vi "Begin.vi"(11 "Image Size":T1=enum."160x120") -> (0 "error out":errorcluster)   [LabVIEW 2012]
doc: "Called before other user functions, this VI is expected to open initial I/O refnums, load in file data, and do all program initialization. Notice that the <B>error out</B> terminal is simply used for data flow. Wiring it to other structures or subVIs ensures that this VI runs first."
uses:
  <vilib>/Rock Robotics/WPI/Camera/WPI_CameraImageSize.ctl
  <vilib>/Rock Robotics/WPI/DriverStation/WPI_DriverStationRobotMode2.ctl
  <vilib>/Rock Robotics/WPI/Joystick/WPI_JoystickDeviceEnum.ctl
  <vilib>/Rock Robotics/WPI/CAN/Jaguar/SubVIs/WPI_CANJaguar_ControlMode.ctl
  <vilib>/Rock Robotics/WPI/CAN/Jaguar/SubVIs/WPI_CANJaguar_SpeedReference.ctl
  <vilib>/Rock Robotics/WPI/CAN/Jaguar/SubVIs/WPI_CANJaguar_BrakeCoastMode.ctl
  <vilib>/Rock Robotics/WPI/CAN/Jaguar/SubVIs/WPI_CANJaguar_PositionReference.ctl
  <vilib>/Rock Robotics/SystemInterfaces/Typedef/FPGA_TypedefDigitalModule.ctl
  <vilib>/Rock Robotics/SystemInterfaces/DIO/FPGA_DIOChannel.ctl
  <vilib>/Rock Robotics/SystemInterfaces/Typedef/FPGA_TypedefSolenoidModule.ctl
  <vilib>/Rock Robotics/WPI/Solenoid/WPI_SolenoidChannel.ctl
  <vilib>/Rock Robotics/SystemInterfaces/DIO/FPGA_DIORelayChannel.ctl
  Robot Global Data.vi
  <vilib>/Rock Robotics/WPI/MotorControl/WPI_MotorControlOpenCANJaguar.vi
  <vilib>/Rock Robotics/WPI/Solenoid/WPI_SolenoidOpenSingle.vi
  <vilib>/Rock Robotics/WPI/Compressor/WPI_CompressorGetSetRefNum.vi
  <vilib>/Rock Robotics/WPI/Camera/WPI_CameraWhite Balance Values.ctl
  <vilib>/Rock Robotics/WPI/Camera/WPI_CameraExposure Values.ctl
  <vilib>/Rock Robotics/WPI/Camera/WPI_CameraFrameRate.ctl
  <vilib>/Rock Robotics/WPI/RobotDrive/WPI_RobotDriveOpen4MotorWithCANJaguar.vi
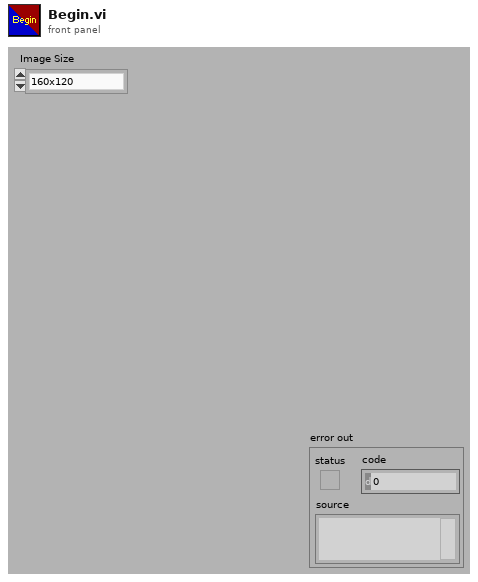
[diagram p1: front panel]
types:
  T1 = typedef "WPI_CameraImageSize.ctl" = enum16{"640x480", "320x240", "160x120"}
  T2 = typedef "FPGA_DIORelayChannel.ctl" = enum8{"Relay 1", "Relay 2", "Relay 3", "Relay 4", "Relay 5", "Relay 6", "Relay 7", "Relay 8", "Invalid"}
  T3 = typedef "WPI_SolenoidChannel.ctl" = enum8{"Solenoid 1", "Solenoid 2", "Solenoid 3", "Solenoid 4", "Solenoid 5", "Solenoid 6", "Solenoid 7", "Solenoid 8", "Invalid"}
  T4 = typedef "FPGA_TypedefSolenoidModule.ctl" = enum16{"Solenoid Module 1", "Solenoid Module 2"}
  T5 = typedef "FPGA_DIOChannel.ctl" = enum8{"DIO 1", "DIO 2", "DIO 3", "DIO 4", "DIO 5", "DIO 6", "DIO 7", "DIO 8", "DIO 9", "DIO 10", "DIO 11", "DIO 12", "DIO 13", "DIO 14", "Invalid"}
  T6 = typedef "FPGA_TypedefDigitalModule.ctl" = enum16{"Digital Module 1", "Digital Module 2"}
  T7 = typedef "WPI_JoystickDeviceEnum.ctl" = enum16{"USB 1", "USB 2", "USB 3", "USB 4", "Kinect 1", "Kinect 2"}
  T8 = typedef "WPI_CANJaguar_PositionReference.ctl" = u8
  T9 = typedef "WPI_CANJaguar_BrakeCoastMode.ctl" = enum8{"Jumper", "Brake", "Coast"}
  T10 = typedef "WPI_CANJaguar_ControlMode.ctl" = enum8{"Percent VBus", "Current", "Speed", "Position", "Voltage"}
  T11 = typedef "WPI_CANJaguar_SpeedReference.ctl" = u8
  T12 = typedef "WPI_DriverStationRobotMode2.ctl" = enum16{"Autonomous Disabled", "Autonomous Enabled", "Teleop Disabled", "Teleop Enabled", "Timeout", "Finish", "Test Disabled", "Test Enabled"}
  T13 = typedef "WPI_JoystickDevRef.ctl" = cluster{"Device":T7}
  T14 = typedef "WPI_SolenoidDevRef.ctl" = cluster{"DevStatus":errorcluster, "Solenoid Module":T4, "Forward Solenoid Channel":T3, "Reverse Solenoid Channel":T3}
  T15 = typedef "WPI_DigitalInputDevRef.ctl" = cluster{"DevStatus":errorcluster, "DIO Channel":T5, "Digital Module":T6}
  T16 = typedef "WPI_CompressorDevRef.ctl" = cluster{"DevStatus":errorcluster, "DigitalInputDevRef":T15, "RelayDevRef":T17}
  T17 = typedef "WPI_RelayDevRef.ctl" = cluster{"DevStatus":errorcluster, "Relay Channel":T2, "Digital Module":T6, "Relay Direction":T18}
  T18 = typedef "WPI_RelayDirection.ctl" = enum16{"Both directions", "Forward only", "Reverse only"}
  T19 = typedef "WPI_SerialPortRef.ctl" = cluster{"DevStatus":errorcluster, "Serial Port Name":refnum<visa-resource-name>}
  T20 = typedef "WPI_CameraFrameRate.ctl" = u32
  T21 = typedef "WPI_CameraExposure Values.ctl" = enum16{"Auto", "Flicker-free 50 Hz", "Flicker-free 60 Hz", "Hold current"}
  T22 = typedef "WPI_CameraWhite Balance Values.ctl" = enum16{"Auto", "Fixed indoor", "Fixed outdoor 1", "Fixed outdoor 2", "Fixed fluorescent 1", "Fixed fluorescent 2", "Hold current"}
  T23 = typedef "WPI_CameraDevRef.ctl" = cluster{"Camera Address":string, "CameraStatus":errorcluster, "Acquire Image Notifier":refnum<notifier>}
  T24 = typedef "WPI_MotorControlDeviceRef.ctl" = cluster{"DeviceStatus":errorcluster, "Type":enum16{"PWM", "CAN"}, "PWM":cluster{"Digital Module":T6, "PWM Channel":T25, "DeadBand":T26}, "CAN":cluster{"Device Number":u8, "Control Mode":T10, "Semaphore":T27, "Max Vout":dbl}, "Invert":bool, "TransformRef":T28, "InvTransformRef":T28}
  T25 = typedef "FPGA_DIOPWMChannel.ctl" = enum8{"PWM 1", "PWM 2", "PWM 3", "PWM 4", "PWM 5", "PWM 6", "PWM 7", "PWM 8", "PWM 9", "PWM 10", "Invalid"}
  T26 = typedef "WPI_PWMDeadband.ctl" = cluster{"Name":string, "maxPositivePwm":i32, "minPositivePwm":i32, "centerPwm":i32, "maxNegativePwm":i32, "minNegativePwm":i32, "angularRange":u16}
  T27 = typedef "Semaphore RefNum" = refnum<k1>
  T28 = typedef "WPI_PWMTransform_ConPane.ctl" = refnum<vi>
  T29 = typedef "WPI_RobotDriveDevRef.ctl" = cluster{"DevStatus":errorcluster, "Motors[]":T24[], "Square Inputs":bool, "Max Output":dbl, "Isochronous":bool}
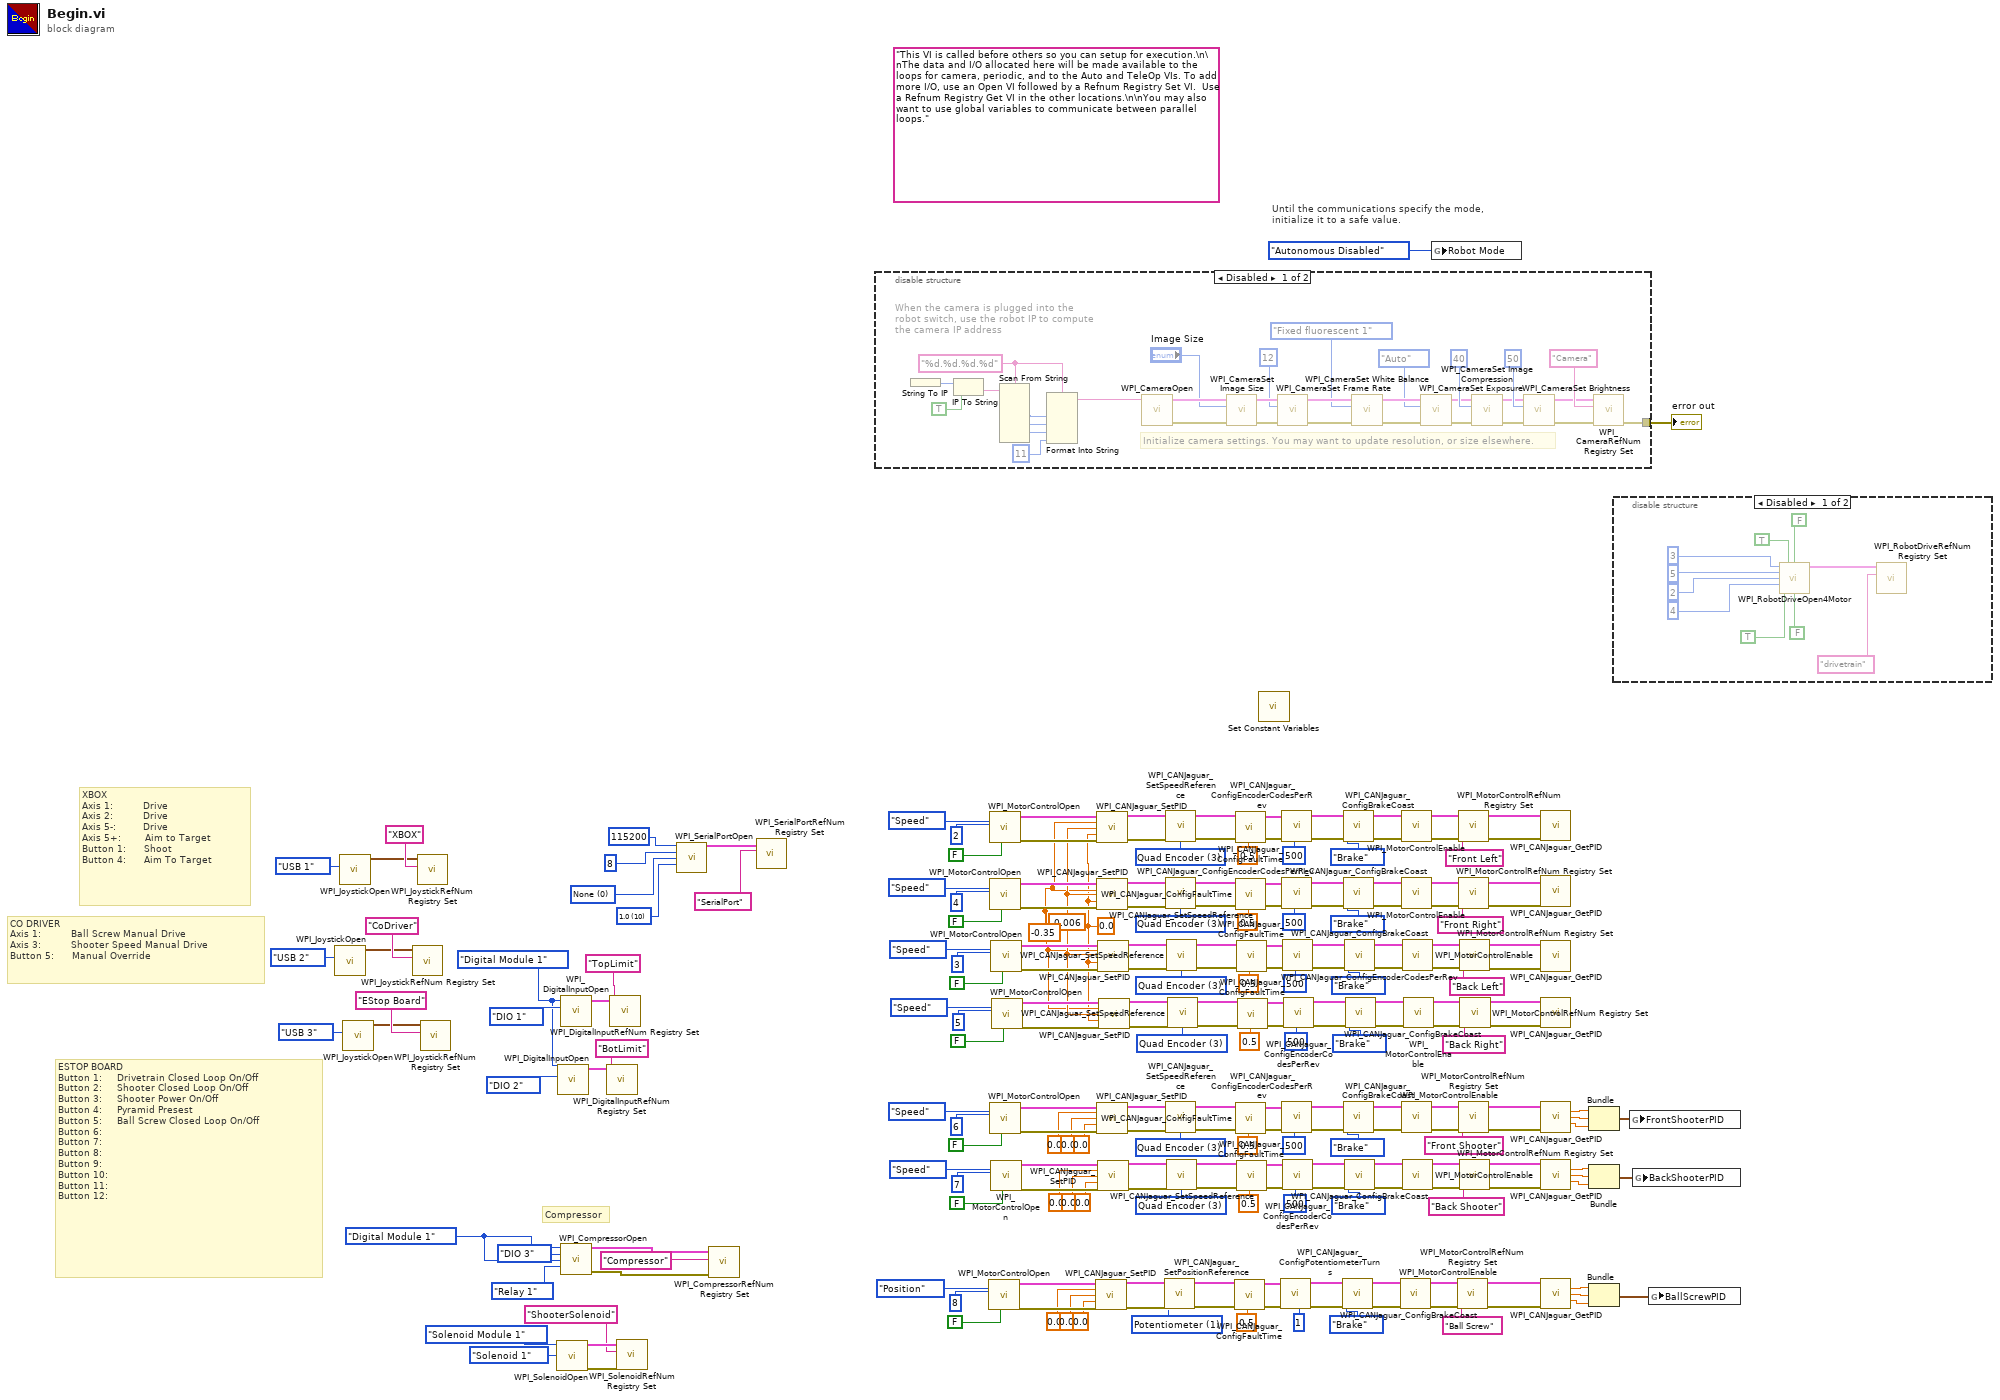
[diagram p0: block diagram]
diagram:
  w2 = FPGA_TypedefDigitalModule."Digital Module 1" ("Pressure Switch Digital Module (Module 1)")
  w12 = FPGA_TypedefDigitalModule."Digital Module 1" ("Digital Module (Module 1)")
  w54 = T8 1 items=["Quad Encoder"=0, "Potentiometer"=1, "None"=255] ("Position Reference")
  w93 = T11 3 items=["Encoder"=0, "Inv Encoder"=2, "Quad Encoder"=3, "None"=255] ("Speed Reference")
  w118 = T11 3 items=["Encoder"=0, "Inv Encoder"=2, "Quad Encoder"=3, "None"=255] ("Speed Reference")
  w140 = T11 3 items=["Encoder"=0, "Inv Encoder"=2, "Quad Encoder"=3, "None"=255] ("Speed Reference")
  w162 = T11 3 items=["Encoder"=0, "Inv Encoder"=2, "Quad Encoder"=3, "None"=255] ("Speed Reference")
  w184 = T11 3 items=["Encoder"=0, "Inv Encoder"=2, "Quad Encoder"=3, "None"=255] ("Speed Reference")
  w20 = -0.35 ("P")
  w21 = -0.006 ("I")
  w19 = 0.0 ("D")
  w206 = T11 3 items=["Encoder"=0, "Inv Encoder"=2, "Quad Encoder"=3, "None"=255] ("Speed Reference")
  w219 = u16 10 items=["1.0"=10, "1.5"=15, "2.0"=20] ("Stop Bits")
  w220 = u16 0 items=["None", "Odd", "Even", "Mark", "Space"] ("Parity")
  (unwired) "This VI is called before others so you can setup for execution.\n\nThe data and I/O allocated here will be made available to the loops for camera, periodic, and to the Auto and TeleOp VIs. To add more I/O, use an Open VI followed by a Refnum Registry Set VI.  Use a Refnum Registry Get VI in the other locations.\n\nYou may also want to use global variables to communicate between parallel loops."
  # "Compressor"
  # "CO DRIVER\nAxis 1:          Ball Screw Manual Drive\nAxis 3:          Shooter Speed Manual Drive\nButton 5:      Manual Override"
  # "XBOX\nAxis 1:          Drive\nAxis 2:          Drive\nAxis 5-:         Drive\nAxis 5+:        Aim to Target\nButton 1:      Shoot\nButton 4:      Aim To Target"
  # "ESTOP BOARD\nButton 1:     Drivetrain Closed Loop On/Off\nButton 2:     Shooter Closed Loop On/Off\nButton 3:     Shooter Power On/Off\nButton 4:     Pyramid Presest\nButton 5:     Ball Screw Closed Loop On/Off\nButton 6:     \nButton 7:\nButton 8:\nButton 9:\nButton 10:\nButton 11:\nButton 12:"
  # "Until the communications specify the mode,\ninitialize it to a safe value."
  n1 = call <vilib>:"WPI_JoystickOpen.vi"("JoystickDevice"=WPI_JoystickDeviceEnum."USB 2") -> ("JoystickDevRef"=w26:T13)  [unwired: 10 in]
  n2 = call <vilib>:"WPI_JoystickOpen.vi"("JoystickDevice"=WPI_JoystickDeviceEnum."USB 1") -> ("JoystickDevRef"=w225:T13)  [unwired: 10 in]
  n3 = call <vilib>:"WPI_JoystickOpen.vi"("JoystickDevice"=WPI_JoystickDeviceEnum."USB 3") -> ("JoystickDevRef"=w23:T13)  [unwired: 10 in]
  n4 = call <vilib>:"WPI_JoystickRefNum Registry Set.vi"("refnum name"="CoDriver", "JoystickDevRef"=w26) -> ()  [unwired: 8 in, 2 out]
  n5 = call <vilib>:"WPI_JoystickRefNum Registry Set.vi"("refnum name"="XBOX", "JoystickDevRef"=w225) -> ()  [unwired: 8 in, 2 out]
  n6 = call <vilib>:"WPI_JoystickRefNum Registry Set.vi"("refnum name"="EStop Board", "JoystickDevRef"=w23) -> ()  [unwired: 8 in, 2 out]
  n7 = call-poly <vilib>:"WPI_SolenoidOpen.vi"("Solenoid Channel"=WPI_SolenoidChannel."Solenoid 1", "Solenoid Module (Module 1)"=FPGA_TypedefSolenoidModule."Solenoid Module 1") -> ("error out"=w5:errorcluster, "SolenoidDevRef"=w4:T14)  [unwired: 8 in]
  n8 = call <vilib>:"WPI_DigitalInputOpen.vi"("DIO Channel"=FPGA_DIOChannel."DIO 2", "Digital Module (Module 1)"=w12) -> ("DigitalInputDevRef"=w15:T15)  [unwired: 8 in, 1 out]
  n9 = call <vilib>:"WPI_DigitalInputOpen.vi"("DIO Channel"=FPGA_DIOChannel."DIO 1", "Digital Module (Module 1)"=w12) -> ("DigitalInputDevRef"=w18:T15)  [unwired: 8 in, 1 out]
  n10 = call <vilib>:"WPI_CompressorOpen.vi"("Pressure Switch Digital Module (Module 1)"=w2, "Pressure Switch DIO Channel"=FPGA_DIOChannel."DIO 3", "Relay Digital Module (Module 1)"=w2, "Relay Channel"=FPGA_DIORelayChannel."Relay 1") -> ("CompressorDevRef"=w9:T16, "error out"=w10:errorcluster)  [unwired: 10 in]
  n11 = call <vilib>:"WPI_DigitalInputRefNum Registry Set.vi"("refnum name"="BotLimit", "DigitalInputDevRef"=w15) -> ()  [unwired: 8 in, 2 out]
  n12 = call <vilib>:"WPI_DigitalInputRefNum Registry Set.vi"("refnum name"="TopLimit", "DigitalInputDevRef"=w18) -> ()  [unwired: 8 in, 2 out]
  n13 = call <vilib>:"WPI_SolenoidRefNum Registry Set.vi"("error in (no error)"=w5, "refnum name"="ShooterSolenoid", "SolenoidDevRef"=w4) -> ()  [unwired: 7 in, 2 out]
  n14 = call <vilib>:"WPI_SerialPortOpen.vi"("Baud Rate"=u32 115200, "Data Bits"=u16 8, "Parity"=w220, "Stop Bits"=w219) -> ("SerialPortRef"=w218:T19)  [unwired: 10 in, 1 out]
  n15 = call <vilib>:"WPI_CompressorRefNum Registry Set.vi"("error in (no error)"=w10, "refnum name"="Compressor", "CompressorDevRef"=w9) -> ()  [unwired: 7 in, 2 out]
  n16 = call <vilib>:"WPI_SerialPortRefNum Registry Set.vi"("refnum name"="SerialPort", "SerialPortRef"=w218) -> ()  [unwired: 8 in, 2 out]
  n17 = disable-structure shown="Disabled" {
    disable-tunnel: [w228 _] -> w223
    frame Disabled {
      w230 = "%d.%d.%d.%d" ("format string")
      # "When the camera is plugged into the\nrobot switch, use the robot IP to compute\nthe camera IP address"
      # "Initialize camera settings. You may want to update resolution, or size elsewhere."
      n18 = String To IP() -> (0:w237:u32)  [unwired: 1 in]
      n19 = IP To String(1:TRUE ("dot notation? (F)"), 2:w237) -> (0:w235:string)
      n20 = Scan From String(format string=w230, input string=w235) -> (output 1=w234:i32, output 2=w233:i32, output 3=w232:i32)  [unwired: 7 in, 3 out]
      n21 = Format Into String(format string=w230, w234, w233, w232, 11 ("Compression")) -> (resulting string=w229:string)  [unwired: 2 in, 1 out]
      n22 = call <vilib>:"WPI_CameraOpen.vi"("Camera Address"=w229) -> ("error out"=w249:errorcluster, "CameraDevRef"=w250:T23)  [unwired: 1 in, 8 out]
      n23 = call <vilib>:"WPI_CameraSet Image Size.vi"("error in (no error)"=w249, "Image Size"="Image Size", "CameraDevRef"=w250) -> ("error out"=w248:errorcluster, "CameraDevRef Out"=w251:T23)  [unwired: 7 out]
      n24 = call <vilib>:"WPI_CameraSet Frame Rate.vi"("error in (no error)"=w248, "Frame Rate (fps)"=T20 12, "CameraDevRef"=w251) -> ("error out"=w247:errorcluster, "CameraDevRef Out"=w253:T23)  [unwired: 7 out]
      n25 = call <vilib>:"WPI_CameraSet White Balance.vi"("error in (no error)"=w247, "White Balance"=WPI_CameraWhite_Balance_Values."Fixed fluorescent 1", "CameraDevRef"=w253) -> ("error out"=w246:errorcluster, "CameraDevRef Out"=w252:T23)  [unwired: 7 out]
      n26 = call <vilib>:"WPI_CameraSet Exposure.vi"("error in (no error)"=w246, "Exposure"=WPI_CameraExposure_Values."Auto", "CameraDevRef"=w252) -> ("error out"=w245:errorcluster, "CameraDevRef Out"=w255:T23)  [unwired: 7 out]
      n27 = call <vilib>:"WPI_CameraSet Image Compression.vi"("error in (no error)"=w245, "Compression"=40, "CameraDevRef"=w255) -> ("error out"=w244:errorcluster, "CameraDevRef Out"=w254:T23)  [unwired: 7 out]
      n28 = call <vilib>:"WPI_CameraSet Brightness.vi"("error in (no error)"=w244, "Brightness"=50, "CameraDevRef"=w254) -> ("error out"=w242:errorcluster, "CameraDevRef Out"=w243:T23)  [unwired: 7 out]
      n29 = call <vilib>:"WPI_CameraRefNum Registry Set.vi"("error in (no error)"=w242, "refnum name"="Camera", "CameraDevRef"=w243) -> ("error out"=w228:errorcluster)  [unwired: 8 out]
    }
    frame Enabled {
    }
  }
  "error out" <- w223
  n30 = call-poly <vilib>:"WPI_MotorControlOpen.vi"("Invert"=FALSE, "Device Number"=u8 8, "Control Mode"=WPI_CANJaguar_ControlMode."Position") -> ("error out"=w72:errorcluster, "MotorControlDeviceRef"=w71:T24)  [unwired: 7 in]
  n31 = call-poly <vilib>:"WPI_MotorControlOpen.vi"("Invert"=FALSE, "Device Number"=u8 2, "Control Mode"=WPI_CANJaguar_ControlMode."Speed") -> ("error out"=w210:errorcluster, "MotorControlDeviceRef"=w209:T24)  [unwired: 7 in]
  n32 = call-poly <vilib>:"WPI_MotorControlOpen.vi"("Invert"=FALSE, "Device Number"=u8 4, "Control Mode"=WPI_CANJaguar_ControlMode."Speed") -> ("error out"=w188:errorcluster, "MotorControlDeviceRef"=w187:T24)  [unwired: 7 in]
  n33 = call-poly <vilib>:"WPI_MotorControlOpen.vi"("Invert"=FALSE, "Device Number"=u8 6, "Control Mode"=WPI_CANJaguar_ControlMode."Speed") -> ("error out"=w122:errorcluster, "MotorControlDeviceRef"=w121:T24)  [unwired: 7 in]
  n34 = call-poly <vilib>:"WPI_MotorControlOpen.vi"("Invert"=FALSE, "Device Number"=u8 3, "Control Mode"=WPI_CANJaguar_ControlMode."Speed") -> ("error out"=w166:errorcluster, "MotorControlDeviceRef"=w165:T24)  [unwired: 7 in]
  n35 = call-poly <vilib>:"WPI_MotorControlOpen.vi"("Invert"=FALSE, "Device Number"=u8 7, "Control Mode"=WPI_CANJaguar_ControlMode."Speed") -> ("error out"=w97:errorcluster, "MotorControlDeviceRef"=w96:T24)  [unwired: 7 in]
  n36 = call-poly <vilib>:"WPI_MotorControlOpen.vi"("Invert"=FALSE, "Device Number"=u8 5, "Control Mode"=WPI_CANJaguar_ControlMode."Speed") -> ("error out"=w144:errorcluster, "MotorControlDeviceRef"=w143:T24)  [unwired: 7 in]
  n37 = call <vilib>:"WPI_CANJaguar_SetPID.vi"("CAN Jaguar Ref"=w71, "P"=0.0, "I"=0.0, "D"=0.0, "error in (no error)"=w72) -> ("CAN Jaguar Ref Out"=w78:T24, "error out"=w77:errorcluster)  [unwired: 9 in]
  n38 = call <vilib>:"WPI_CANJaguar_SetPID.vi"("CAN Jaguar Ref"=w209, "P"=w20, "I"=w21, "D"=w19, "error in (no error)"=w210) -> ("CAN Jaguar Ref Out"=w216:T24, "error out"=w215:errorcluster)  [unwired: 9 in]
  n39 = call <vilib>:"WPI_CANJaguar_SetPID.vi"("CAN Jaguar Ref"=w187, "P"=w20, "I"=w21, "D"=w19, "error in (no error)"=w188) -> ("CAN Jaguar Ref Out"=w194:T24, "error out"=w193:errorcluster)  [unwired: 9 in]
  n40 = call <vilib>:"WPI_CANJaguar_SetPID.vi"("CAN Jaguar Ref"=w121, "P"=0.0, "I"=0.0, "D"=0.0, "error in (no error)"=w122) -> ("CAN Jaguar Ref Out"=w128:T24, "error out"=w127:errorcluster)  [unwired: 9 in]
  n41 = call <vilib>:"WPI_CANJaguar_SetPID.vi"("CAN Jaguar Ref"=w165, "P"=w20, "I"=w21, "D"=w19, "error in (no error)"=w166) -> ("CAN Jaguar Ref Out"=w172:T24, "error out"=w171:errorcluster)  [unwired: 9 in]
  n42 = call <vilib>:"WPI_CANJaguar_SetPID.vi"("CAN Jaguar Ref"=w96, "P"=0.0, "I"=0.0, "D"=0.0, "error in (no error)"=w97) -> ("CAN Jaguar Ref Out"=w103:T24, "error out"=w102:errorcluster)  [unwired: 9 in]
  n43 = call <vilib>:"WPI_CANJaguar_SetPID.vi"("CAN Jaguar Ref"=w143, "P"=w20, "I"=w21, "D"=w19, "error in (no error)"=w144) -> ("CAN Jaguar Ref Out"=w150:T24, "error out"=w149:errorcluster)  [unwired: 9 in]
  n44 = call <vilib>:"WPI_CANJaguar_SetPositionReference.vi"("error in (no error)"=w77, "Position Reference"=w54, "CAN Jaguar Ref"=w78) -> ("error out"=w76:errorcluster, "CAN Jaguar Ref Out"=w75:T24)  [unwired: 7 in]
  n45 = call <vilib>:"WPI_CANJaguar_SetSpeedReference.vi"("error in (no error)"=w215, "Speed Reference"=w206, "CAN Jaguar Ref"=w216) -> ("error out"=w214:errorcluster, "CAN Jaguar Ref Out"=w213:T24)  [unwired: 7 in]
  n46 = call <vilib>:"WPI_CANJaguar_SetSpeedReference.vi"("error in (no error)"=w193, "Speed Reference"=w184, "CAN Jaguar Ref"=w194) -> ("error out"=w192:errorcluster, "CAN Jaguar Ref Out"=w191:T24)  [unwired: 7 in]
  n47 = call <vilib>:"WPI_CANJaguar_SetSpeedReference.vi"("error in (no error)"=w127, "Speed Reference"=w118, "CAN Jaguar Ref"=w128) -> ("error out"=w126:errorcluster, "CAN Jaguar Ref Out"=w125:T24)  [unwired: 7 in]
  n48 = call <vilib>:"WPI_CANJaguar_SetSpeedReference.vi"("error in (no error)"=w171, "Speed Reference"=w162, "CAN Jaguar Ref"=w172) -> ("error out"=w170:errorcluster, "CAN Jaguar Ref Out"=w169:T24)  [unwired: 7 in]
  n49 = call <vilib>:"WPI_CANJaguar_SetSpeedReference.vi"("error in (no error)"=w102, "Speed Reference"=w93, "CAN Jaguar Ref"=w103) -> ("error out"=w101:errorcluster, "CAN Jaguar Ref Out"=w100:T24)  [unwired: 7 in]
  n50 = call <vilib>:"WPI_CANJaguar_SetSpeedReference.vi"("error in (no error)"=w149, "Speed Reference"=w140, "CAN Jaguar Ref"=w150) -> ("error out"=w148:errorcluster, "CAN Jaguar Ref Out"=w147:T24)  [unwired: 7 in]
  n51 = call <vilib>:"WPI_CANJaguar_ConfigFaultTime.vi"("error in (no error)"=w76, "Fault Time (s)"=0.5, "CAN Jaguar Ref"=w75) -> ("error out"=w73:errorcluster, "CAN Jaguar Ref Out"=w74:T24)  [unwired: 7 in]
  n52 = call <vilib>:"WPI_CANJaguar_ConfigFaultTime.vi"("error in (no error)"=w214, "Fault Time (s)"=0.5, "CAN Jaguar Ref"=w213) -> ("error out"=w211:errorcluster, "CAN Jaguar Ref Out"=w212:T24)  [unwired: 7 in]
  n53 = call <vilib>:"WPI_CANJaguar_ConfigFaultTime.vi"("error in (no error)"=w192, "Fault Time (s)"=0.5, "CAN Jaguar Ref"=w191) -> ("error out"=w189:errorcluster, "CAN Jaguar Ref Out"=w190:T24)  [unwired: 7 in]
  n54 = call <vilib>:"WPI_CANJaguar_ConfigFaultTime.vi"("error in (no error)"=w126, "Fault Time (s)"=0.5, "CAN Jaguar Ref"=w125) -> ("error out"=w123:errorcluster, "CAN Jaguar Ref Out"=w124:T24)  [unwired: 7 in]
  n55 = call <vilib>:"WPI_CANJaguar_ConfigFaultTime.vi"("error in (no error)"=w170, "Fault Time (s)"=0.5, "CAN Jaguar Ref"=w169) -> ("error out"=w167:errorcluster, "CAN Jaguar Ref Out"=w168:T24)  [unwired: 7 in]
  n56 = call <vilib>:"WPI_CANJaguar_ConfigFaultTime.vi"("error in (no error)"=w101, "Fault Time (s)"=0.5, "CAN Jaguar Ref"=w100) -> ("error out"=w98:errorcluster, "CAN Jaguar Ref Out"=w99:T24)  [unwired: 7 in]
  n57 = call <vilib>:"WPI_CANJaguar_ConfigFaultTime.vi"("error in (no error)"=w148, "Fault Time (s)"=0.5, "CAN Jaguar Ref"=w147) -> ("error out"=w145:errorcluster, "CAN Jaguar Ref Out"=w146:T24)  [unwired: 7 in]
  n58 = call "Set Constant Variables.vi"() -> ()  [unwired: 12 in]
  n59 = call <vilib>:"WPI_CANJaguar_ConfigPotentiometerTurns.vi"("error in (no error)"=w73, "Potentiometer Turns"=u16 1 ("Encoder Codes Per Rev"), "CAN Jaguar Ref"=w74) -> ("error out"=w66:errorcluster, "CAN Jaguar Ref Out"=w65:T24)  [unwired: 7 in]
  n60 = call <vilib>:"WPI_CANJaguar_ConfigEncoderCodesPerRev.vi"("error in (no error)"=w211, "Encoder Codes Per Rev"=u16 500, "CAN Jaguar Ref"=w212) -> ("error out"=w203:errorcluster, "CAN Jaguar Ref Out"=w202:T24)  [unwired: 7 in]
  n61 = call <vilib>:"WPI_CANJaguar_ConfigEncoderCodesPerRev.vi"("error in (no error)"=w189, "Encoder Codes Per Rev"=u16 500, "CAN Jaguar Ref"=w190) -> ("error out"=w181:errorcluster, "CAN Jaguar Ref Out"=w180:T24)  [unwired: 7 in]
  n62 = call <vilib>:"WPI_CANJaguar_ConfigEncoderCodesPerRev.vi"("error in (no error)"=w123, "Encoder Codes Per Rev"=u16 500, "CAN Jaguar Ref"=w124) -> ("error out"=w115:errorcluster, "CAN Jaguar Ref Out"=w114:T24)  [unwired: 7 in]
  n63 = call <vilib>:"WPI_CANJaguar_ConfigEncoderCodesPerRev.vi"("error in (no error)"=w167, "Encoder Codes Per Rev"=u16 500, "CAN Jaguar Ref"=w168) -> ("error out"=w159:errorcluster, "CAN Jaguar Ref Out"=w158:T24)  [unwired: 7 in]
  n64 = call <vilib>:"WPI_CANJaguar_ConfigEncoderCodesPerRev.vi"("error in (no error)"=w98, "Encoder Codes Per Rev"=u16 500, "CAN Jaguar Ref"=w99) -> ("error out"=w90:errorcluster, "CAN Jaguar Ref Out"=w89:T24)  [unwired: 7 in]
  n65 = call <vilib>:"WPI_CANJaguar_ConfigEncoderCodesPerRev.vi"("error in (no error)"=w145, "Encoder Codes Per Rev"=u16 500, "CAN Jaguar Ref"=w146) -> ("error out"=w137:errorcluster, "CAN Jaguar Ref Out"=w136:T24)  [unwired: 7 in]
  n66 = call <vilib>:"WPI_CANJaguar_ConfigBrakeCoast.vi"("error in (no error)"=w66, "Brake / Coast Mode"=WPI_CANJaguar_BrakeCoastMode."Brake", "CAN Jaguar Ref"=w65) -> ("error out"=w57:errorcluster, "CAN Jaguar Ref Out"=w58:T24)  [unwired: 7 in]
  n67 = call <vilib>:"WPI_CANJaguar_ConfigBrakeCoast.vi"("error in (no error)"=w203, "Brake / Coast Mode"=WPI_CANJaguar_BrakeCoastMode."Brake", "CAN Jaguar Ref"=w202) -> ("error out"=w197:errorcluster, "CAN Jaguar Ref Out"=w198:T24)  [unwired: 7 in]
  n68 = call <vilib>:"WPI_CANJaguar_ConfigBrakeCoast.vi"("error in (no error)"=w181, "Brake / Coast Mode"=WPI_CANJaguar_BrakeCoastMode."Brake", "CAN Jaguar Ref"=w180) -> ("error out"=w175:errorcluster, "CAN Jaguar Ref Out"=w176:T24)  [unwired: 7 in]
  n69 = call <vilib>:"WPI_CANJaguar_ConfigBrakeCoast.vi"("error in (no error)"=w115, "Brake / Coast Mode"=WPI_CANJaguar_BrakeCoastMode."Brake", "CAN Jaguar Ref"=w114) -> ("error out"=w106:errorcluster, "CAN Jaguar Ref Out"=w107:T24)  [unwired: 7 in]
  n70 = call <vilib>:"WPI_CANJaguar_ConfigBrakeCoast.vi"("error in (no error)"=w159, "Brake / Coast Mode"=WPI_CANJaguar_BrakeCoastMode."Brake", "CAN Jaguar Ref"=w158) -> ("error out"=w153:errorcluster, "CAN Jaguar Ref Out"=w154:T24)  [unwired: 7 in]
  n71 = call <vilib>:"WPI_CANJaguar_ConfigBrakeCoast.vi"("error in (no error)"=w90, "Brake / Coast Mode"=WPI_CANJaguar_BrakeCoastMode."Brake", "CAN Jaguar Ref"=w89) -> ("error out"=w81:errorcluster, "CAN Jaguar Ref Out"=w82:T24)  [unwired: 7 in]
  n72 = call <vilib>:"WPI_CANJaguar_ConfigBrakeCoast.vi"("error in (no error)"=w137, "Brake / Coast Mode"=WPI_CANJaguar_BrakeCoastMode."Brake", "CAN Jaguar Ref"=w136) -> ("error out"=w131:errorcluster, "CAN Jaguar Ref Out"=w132:T24)  [unwired: 7 in]
  n73 = call <vilib>:"WPI_MotorControlEnable.vi"("error in (no error)"=w57, "CAN Jaguar Ref"=w58) -> ("error out"=w55:errorcluster, "CAN Jaguar Ref Out"=w56:T24)  [unwired: 8 in]
  n74 = call <vilib>:"WPI_MotorControlEnable.vi"("error in (no error)"=w197, "CAN Jaguar Ref"=w198) -> ("error out"=w195:errorcluster, "CAN Jaguar Ref Out"=w196:T24)  [unwired: 8 in]
  n75 = call <vilib>:"WPI_MotorControlEnable.vi"("error in (no error)"=w175, "CAN Jaguar Ref"=w176) -> ("error out"=w173:errorcluster, "CAN Jaguar Ref Out"=w174:T24)  [unwired: 8 in]
  n76 = call <vilib>:"WPI_MotorControlEnable.vi"("error in (no error)"=w106, "CAN Jaguar Ref"=w107) -> ("error out"=w104:errorcluster, "CAN Jaguar Ref Out"=w105:T24)  [unwired: 8 in]
  n77 = call <vilib>:"WPI_MotorControlEnable.vi"("error in (no error)"=w153, "CAN Jaguar Ref"=w154) -> ("error out"=w151:errorcluster, "CAN Jaguar Ref Out"=w152:T24)  [unwired: 8 in]
  n78 = call <vilib>:"WPI_MotorControlEnable.vi"("error in (no error)"=w81, "CAN Jaguar Ref"=w82) -> ("error out"=w79:errorcluster, "CAN Jaguar Ref Out"=w80:T24)  [unwired: 8 in]
  n79 = call <vilib>:"WPI_MotorControlEnable.vi"("error in (no error)"=w131, "CAN Jaguar Ref"=w132) -> ("error out"=w129:errorcluster, "CAN Jaguar Ref Out"=w130:T24)  [unwired: 8 in]
  n80 = global write "Robot Global Data.vi" "Robot Mode"(WPI_DriverStationRobotMode2."Autonomous Disabled" ("Robot Mode")) -> ()
  n81 = call <vilib>:"WPI_MotorControlRefNum Registry Set.vi"("error in (no error)"=w55, "refnum name"="Ball Screw", "MotorControlDevRef"=w56) -> ("error out"=w28:errorcluster, "MotorControlDevRef"=w29:T24)  [unwired: 7 in]
  n82 = call <vilib>:"WPI_MotorControlRefNum Registry Set.vi"("error in (no error)"=w195, "refnum name"="Front Left", "MotorControlDevRef"=w196) -> ("error out"=w49:errorcluster, "MotorControlDevRef"=w53:T24)  [unwired: 7 in]
  n83 = call <vilib>:"WPI_MotorControlRefNum Registry Set.vi"("error in (no error)"=w173, "refnum name"="Front Right", "MotorControlDevRef"=w174) -> ("error out"=w50:errorcluster, "MotorControlDevRef"=w51:T24)  [unwired: 7 in]
  n84 = call <vilib>:"WPI_MotorControlRefNum Registry Set.vi"("error in (no error)"=w104, "refnum name"="Front Shooter", "MotorControlDevRef"=w105) -> ("error out"=w32:errorcluster, "MotorControlDevRef"=w33:T24)  [unwired: 7 in]
  n85 = call <vilib>:"WPI_MotorControlRefNum Registry Set.vi"("error in (no error)"=w151, "refnum name"="Back Left", "MotorControlDevRef"=w152) -> ("error out"=w48:errorcluster, "MotorControlDevRef"=w52:T24)  [unwired: 7 in]
  n86 = call <vilib>:"WPI_MotorControlRefNum Registry Set.vi"("error in (no error)"=w79, "refnum name"="Back Shooter", "MotorControlDevRef"=w80) -> ("error out"=w30:errorcluster, "MotorControlDevRef"=w31:T24)  [unwired: 7 in]
  n87 = call <vilib>:"WPI_MotorControlRefNum Registry Set.vi"("error in (no error)"=w129, "refnum name"="Back Right", "MotorControlDevRef"=w130) -> ("error out"=w46:errorcluster, "MotorControlDevRef"=w47:T24)  [unwired: 7 in]
  n88 = call <vilib>:"WPI_CANJaguar_GetPID.vi"("CAN Jaguar Ref"=w53, "error in (no error)"=w49) -> ()  [unwired: 9 in, 5 out]
  n89 = call <vilib>:"WPI_CANJaguar_GetPID.vi"("CAN Jaguar Ref"=w51, "error in (no error)"=w50) -> ()  [unwired: 9 in, 5 out]
  n90 = call <vilib>:"WPI_CANJaguar_GetPID.vi"("CAN Jaguar Ref"=w52, "error in (no error)"=w48) -> ()  [unwired: 9 in, 5 out]
  n91 = call <vilib>:"WPI_CANJaguar_GetPID.vi"("CAN Jaguar Ref"=w47, "error in (no error)"=w46) -> ()  [unwired: 9 in, 5 out]
  n92 = call <vilib>:"WPI_CANJaguar_GetPID.vi"("CAN Jaguar Ref"=w33, "error in (no error)"=w32) -> ("P"=w44:dbl, "I"=w42:dbl, "D"=w43:dbl)  [unwired: 9 in, 2 out]
  n93 = call <vilib>:"WPI_CANJaguar_GetPID.vi"("CAN Jaguar Ref"=w31, "error in (no error)"=w30) -> ("P"=w40:dbl, "I"=w38:dbl, "D"=w39:dbl)  [unwired: 9 in, 2 out]
  n94 = call <vilib>:"WPI_CANJaguar_GetPID.vi"("CAN Jaguar Ref"=w29, "error in (no error)"=w28) -> ("P"=w36:dbl, "I"=w34:dbl, "D"=w35:dbl)  [unwired: 9 in, 2 out]
  n95 = Bundle("P"=w44, "I"=w42, "D"=w43) -> (w45:cluster{"P":dbl, "I":dbl, "D":dbl})  [unwired: 1 in]
  n96 = Bundle("P"=w40, "I"=w38, "D"=w39) -> (w41:cluster{"P":dbl, "I":dbl, "D":dbl})  [unwired: 1 in]
  n97 = Bundle("P"=w36, "I"=w34, "D"=w35) -> (w37:cluster{"P":dbl, "I":dbl, "D":dbl})  [unwired: 1 in]
  n98 = disable-structure shown="Disabled" {
    frame Disabled {
      n99 = call-poly <vilib>:"WPI_RobotDriveOpen4Motor.vi"("Rear Left Motor"=u8 3, "Rear Left Motor Inverted"=TRUE, "Rear Right Motor Inverted"=FALSE, "Rear Right Motor"=u8 5 ("Rear Left Motor"), "Front Left Motor"=u8 2 ("Rear Left Motor"), "Front Right Motor"=u8 4 ("Rear Left Motor"), "Front Left Motor Inverted"=TRUE, "Front Right Motor Inverted"=FALSE) -> ("RobotDriveDevRef"=w260:T29)  [unwired: 6 in, 1 out]
      n100 = call <vilib>:"WPI_RobotDriveRefNum Registry Set.vi"("refnum name"="drivetrain", "RobotDriveDevRef"=w260) -> ()  [unwired: 8 in, 2 out]
    }
    frame Enabled {
    }
  }
  n101 = global write "Robot Global Data.vi" "FrontShooterPID"(w45) -> ()
  n102 = global write "Robot Global Data.vi" "BackShooterPID"(w41) -> ()
  n103 = global write "Robot Global Data.vi" "BallScrewPID"(w37) -> ()
